vi "In-Range Image.vi"   [LabVIEW 2020, in "image.lvlib"]
doc: "Compute a single channel image which will contain non-zero pixels for any pixel in the Source Image which is between the two Pixel Values specified. The range values are interpolated using the HSV colour-space.\n\nThis is similar to Image \"Match-Value\" except it matches between an upper and lower value."
uses:
  image.lvlib
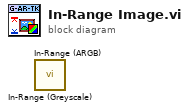
[diagram p0: block diagram]
diagram:
  n1 = call "In-Range (Greyscale).vi"() -> ()  [unwired: 10 in, 2 out]
  n2 = call "In-Range (ARGB).vi"() -> ()  [unwired: 10 in, 2 out]
